vi "GaiaSimulateDUTReplace.vi"(8 "error in":errorcluster, 11 "GaiaClientRef in":refnum<k24>) -> (0 "error out":errorcluster, 3 "GaiaClientRef out":refnum<k24>)   [LabVIEW 2019]
uses:
  C:/GIT/gaialabviewclient/Gaia_LabVIEW/Resources/JOT.GaiaClient.dll
  Resources/JOT.GaiaClient.dll
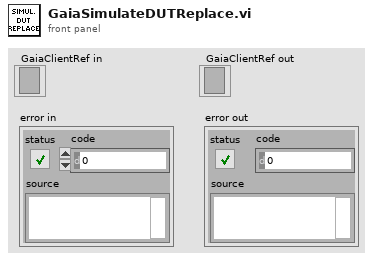
[diagram p1: front panel]
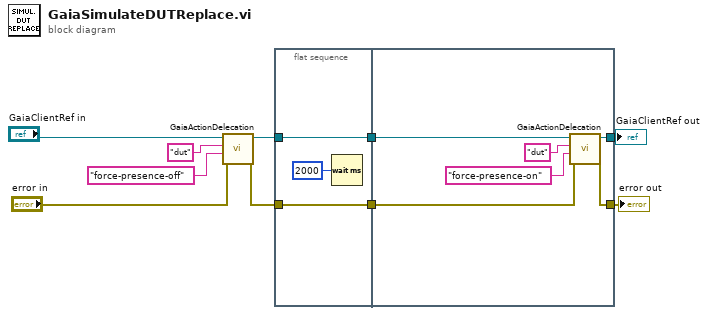
[diagram p0: block diagram]
diagram:
  n1 = call "GaiaActionDelecation.vi"("Error in"="error in", "Action"="force-presence-off", "Application"="dut", "ClientRef"="GaiaClientRef in") -> ("error out"=w6:errorcluster, "ClientRef out"=w9:refnum<k24>)  [unwired: 6 in]
  n2 = flat-sequence {
    tunnel: w6 -> [w12]
    tunnel: w9 -> [w13]
    tunnel: [w13] -> w2
    tunnel: [w12] -> w1
    tunnel: [w18] -> w8
    tunnel: [w17] -> w7
    tunnel: w2 -> [w19]
    tunnel: w1 -> [w16]
    frame #0 {
      n3 = Wait (ms)(milliseconds to wait=u32 2000) -> ()  [unwired: 1 out]
    }
    frame #1 {
      n4 = call "GaiaActionDelecation.vi"("Error in"=w16, "Action"="force-presence-on", "Application"="dut", "ClientRef"=w19) -> ("error out"=w17:errorcluster, "ClientRef out"=w18:refnum<k24>)  [unwired: 6 in]
    }
  }
  "error out" <- w7
  "GaiaClientRef out" <- w8
